vi "NanotecSMCPDDriver.get percent current.vi"(1 "hardwareType":T1) -> (0 "percentCurrent [A/%]":dbl)   [LabVIEW 2014, in "NanotecSMCPDDriver.lvlib"]
doc: "Nanotec controller und plug&play drives allow to set the phase current in percent units, from 0..150. Values above 100% are not recommended. This VI gives the current corresponding to 1% depending on the hardware."
uses:
  NanotecSMCPDDriver.lvlib
  NanotecSMCPDDriver.hardware types.ctl
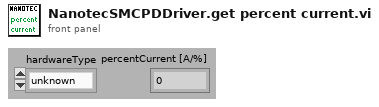
[diagram p1: front panel]
types:
  T1 = typedef "NanotecSMCPDDriver.lvlib/NanotecSMCPDDriver.hardware types.ctl" = enum16{"unknown", "PD4", "PD4Ic", "PD2Ic", "SMCI32", "SMCI47"}
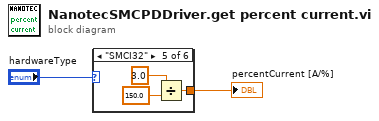
[diagram p0: block diagram]
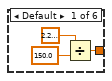
[diagram p2: hidden frame]
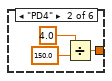
[diagram p3: hidden frame]
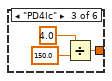
[diagram p4: hidden frame]
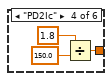
[diagram p5: hidden frame]
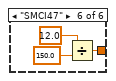
[diagram p6: hidden frame]
diagram:
  n1 = case shown="\"SMCI32\"" "hardwareType" {
    tunnel: [w3 w6 w9 w12 w15 w18] -> w2
    frame Default {
      n2 = Divide(x=2.220446049250313e-16 ("Machine Epsilon"), y=150.0) -> (x/y=w3:dbl)
    }
    frame "PD4" {
      n3 = Divide(x=4.0, y=150.0) -> (x/y=w6:dbl)
    }
    frame "PD4Ic" {
      n4 = Divide(x=4.0, y=150.0) -> (x/y=w9:dbl)
    }
    frame "PD2Ic" {
      n5 = Divide(x=1.8, y=150.0) -> (x/y=w12:dbl)
    }
    frame "SMCI32" {
      n6 = Divide(x=3.0, y=150.0) -> (x/y=w15:dbl)
    }
    frame "SMCI47" {
      n7 = Divide(x=12.0, y=150.0) -> (x/y=w18:dbl)
    }
  }
  "percentCurrent [A/%]" <- w2
